vi "Add_Base_URL.vi"(8 "error in (no error)":errorcluster, 10 "Base URL":string, 11 "Request in":refnum<class "Request.lvclass">) -> (0 "error out":errorcluster, 3 "Request out":refnum<class "Request.lvclass">)   [LabVIEW 2016, in "Request.lvclass"]
uses:
  Request.lvclass
  <vilib>/Utility/error.llb/whitespace.ctl
  Request.lvclass/Request.ctl
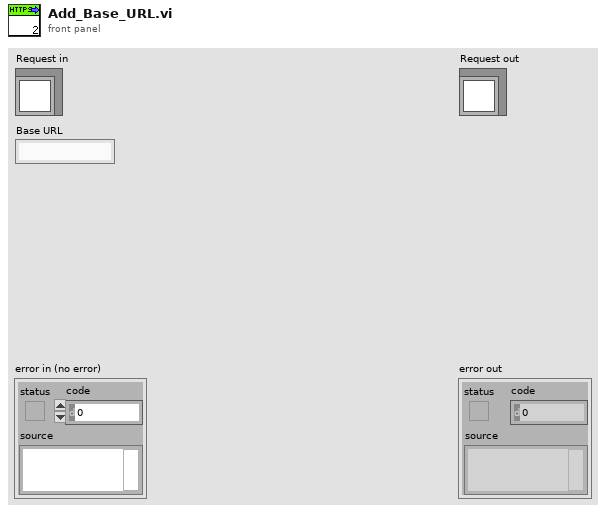
[diagram p1: front panel]
types:
  T1 = typedef "whitespace.ctl" = u16
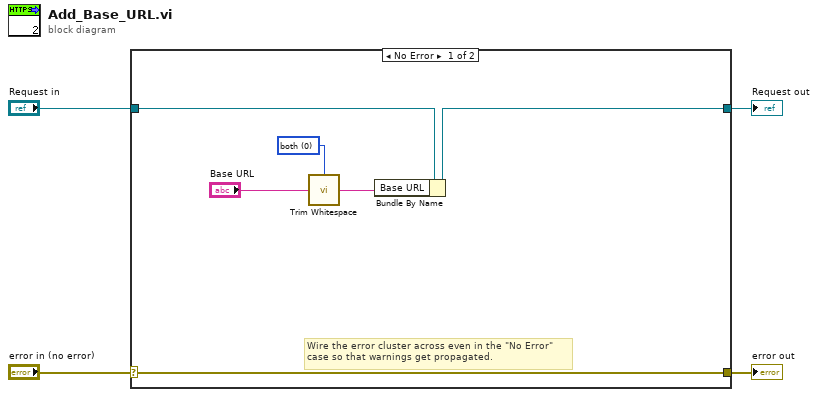
[diagram p0: block diagram]
diagram:
  n1 = case shown="No Error" "error in (no error)" {
    selector: "error in (no error)" -> [w10 w12]
    tunnel: [w10 w12] -> w3
    tunnel: [w8 w11] -> w1
    tunnel: "Request in" -> [w9 w11]
    frame No Error {
      w5 = T1 0 items=["both", "start of string", "end of string"] ("location (both)")
      # "Wire the error cluster across even in the \"No Error\"\ncase so that warnings get propagated."
      n2 = call <vilib>:"Trim Whitespace.vi"("string"="Base URL", "location (both)"=w5) -> ("trimmed string"=w6:string)
      n3 = Bundle By Name(cluster=w9, "Base URL"=w6) -> (w8:refnum<class "Request.lvclass">)
    }
    frame Error {
    }
  }
  "error out" <- w3
  "Request out" <- w1
